vi "Raise Event.vi"(8 "error in (no error)":errorcluster, 10 "EventDataObj":refnum<class "EventData.lvclass">, 11 "Event in":refnum<class "Event.lvclass">) -> (0 "error out":errorcluster, 1 "InvalidEventRef?":bool, 3 "Event out":refnum<class "Event.lvclass">)   [LabVIEW 2021, in "EventManagerLibrary.lvlib" / "Event.lvclass"]
doc: "Raises the event contained in this event object.\n\nThis vi runs normally even if an error occurred before this vi."
uses:
  Event.lvclass
  EventDataObject/EventData.lvclass
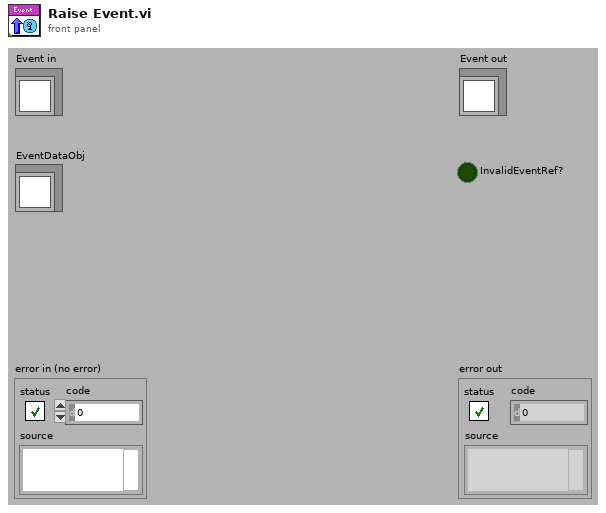
[diagram p1: front panel]
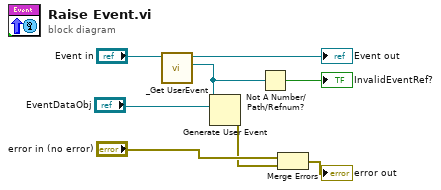
[diagram p0: block diagram]
diagram:
  n1 = call "_Get UserEvent.vi"("Event in"="Event in") -> ("UserEvent"=w4:refnum<user-event>, "Event out"=→"Event out":refnum<class "Event.lvclass">)  [unwired: 1 in, 8 out]
  n2 = Generate User Event(user event=w4, event data cluster="EventDataObj") -> (error out=w2:errorcluster)  [unwired: 2 in, 1 out]
  n3 = Not A Number/Path/Refnum?(number/path/refnum=w4) -> (NaN/Path/Refnum?=→"InvalidEventRef?":bool)
  n4 = Merge Errors("error in (no error)", w2) -> (→"error out":errorcluster)
